vi "Auton Unpack.vi"(5 "all rows":dbl[][](array[numeric]), 9 "Index":i32) -> (0 "Timer":dbl, 1 "Indicate Index":i32, 2 "Right Stick":dbl, 3 "Left Stick":dbl, 4 "Right Drive Power":dbl, 6 "Left Drive Power":dbl, 8 "Right Distance":dbl, 10 "Left Distance":dbl, 12 "Arm":dbl, 13 "Gripper":dbl, 14 "Wrist":dbl, 15 "Auton Status":dbl)   [LabVIEW 2014]
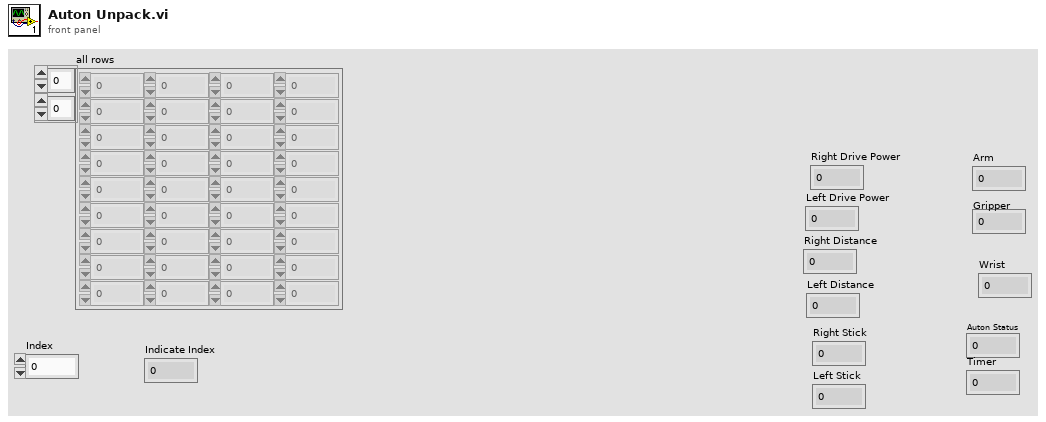
[diagram p1: front panel]
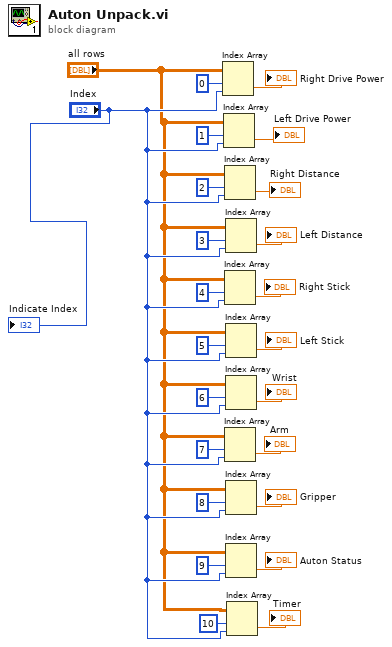
[diagram p0: block diagram]
diagram:
  n1 = Index Array(array="all rows", index (row)=0, index (col)="Index") -> (element=→"Right Drive Power":dbl)
  n2 = Index Array(array="all rows", index (row)=1, index (col)="Index") -> (element=→"Left Drive Power":dbl)
  n3 = Index Array(array="all rows", index (row)=2, index (col)="Index") -> (element=→"Right Distance":dbl)
  n4 = Index Array(array="all rows", index (row)=4, index (col)="Index") -> (element=→"Right Stick":dbl)
  n5 = Index Array(array="all rows", index (row)=7, index (col)="Index") -> (element=→"Arm":dbl)
  n6 = Index Array(array="all rows", index (row)=3, index (col)="Index") -> (element=→"Left Distance":dbl)
  n7 = Index Array(array="all rows", index (row)=5, index (col)="Index") -> (element=→"Left Stick":dbl)
  n8 = Index Array(array="all rows", index (row)=6, index (col)="Index") -> (element=→"Wrist":dbl)
  n9 = Index Array(array="all rows", index (row)=8, index (col)="Index") -> (element=→"Gripper":dbl)
  n10 = Index Array(array="all rows", index (row)=9, index (col)="Index") -> (element=→"Auton Status":dbl)
  n11 = Index Array(array="all rows", index (row)=10, index (col)="Index") -> (element=→"Timer":dbl)
  "Indicate Index" <- "Index"
